vi "pickRobotsVSS.vi"(8 "error in (no error)":errorcluster, 11 "Game in":refnum<class "Game.lvclass">) -> (0 "error out":errorcluster, 3 "Game out":refnum<class "Game.lvclass">)   [LabVIEW 2018, in "Game.lvclass"]
uses:
  Game.lvclass
  Game.lvclass/Game.ctl
  Referee_class/Referee.lvclass/Referee.ctl
  Team_class/Team.lvclass/Team.ctl
  Robot_class/roles.ctl
  Robot_class/Robot.lvclass/Robot.ctl
  Role_class/Role.lvclass/Role.ctl
  HaltPlay_class/HaltPlay.lvclass/HaltPlay.ctl
  Playbook_class/Playbook.lvclass/Playbook.ctl
  ZigZagPlay_class/ZigZagPlay.lvclass/ZigZagPlay.ctl
  Robot_class/Robot.lvclass
  Playbook_class/Playbook.lvclass
  Ally_class/Ally.lvclass
  C:/Users/anton/Desktop/RoboIme/vsspssl/SSL_AI/Team_class/Team.lvclass
  Role_class/Write RobotRef.vi
  Robot_class/Write role.vi
  HaltPlay_class/Read Roles.vi
  HaltPlay_class/Write Roles.vi
  ZigZagPlay_class/Read Roles.vi
  ZigZagPlay_class/Write Roles.vi
  Playbook_class/Write keeper_plays.vi
  Playbook_class/Read keeper_plays.vi
  Read KeeperTeam.vi
  Read AllyRef.vi
  Read Referee.vi
  Read TestMode IDs.vi
  Referee_class/Read our_goalie_id.vi
  Team_class/Read RobotRef.vi
  Team_class/Write RobotRef.vi
  Write KeeperTeam.vi
  TimeoutRole_class/TimeoutRole.lvclass
  C:/Users/anton/Desktop/RoboIme/vsspssl/SSL_AI/Role_class/Role.lvclass
  HaltRole_class/HaltRole.lvclass
  ZigZagRole_class/ZigZagRole.lvclass
  Referee_class/Referee.lvclass
  PreparePenaltyAllyPlayVSS_class/PreparePenaltyAllyPlayVSS.lvclass
  HaltPlay_class/HaltPlay.lvclass
  DeadBallPlayVSS_class/DeadBallPlayVSS.lvclass
  NormalGamePlayVSS_class/NormalGamePlayVSS.lvclass
  BallChallengePlayVSS_class/BallChallengePlayVSS.lvclass
  PenaltyEnemyPlayVSS_class/PenaltyEnemyPlayVSS.lvclass
  TimeoutPlay_class/TimeoutPlay.lvclass
  Play_class/Play.lvclass
  TestPlay_class/TestPlay.lvclass
  KeeperPlay_class/KeeperPlay.lvclass
  ZigZagPlay_class/ZigZagPlay.lvclass
  GoToPlay_class/GoToPlay.lvclass
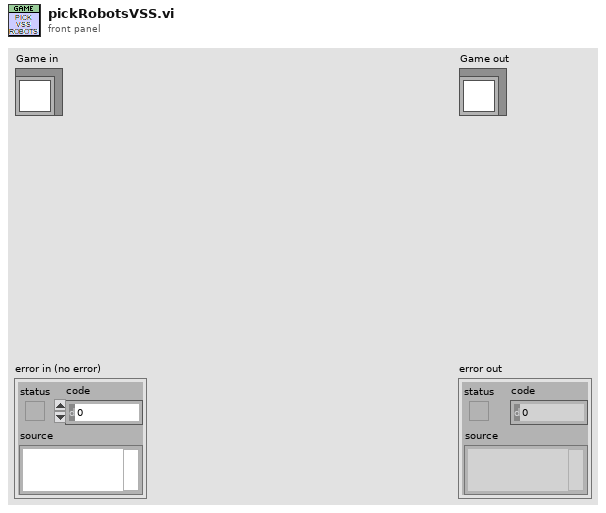
[diagram p1: front panel]
types:
  T1 = typedef "roles.ctl" = enum16{"Tabler", "TableFinalizer", "PrepareRollToPassRoller", "PrepareRollToPassReceiver", "SimplePassRoll", "SimplePassRollReceiver", "PenaltyDefense", "PreparePassReceiver 2", "PreparePassReceiver 1", "PassObserver", "Timeout", "Goto", "ZigZag", "None", "BallOutOfField", "DefenderArea", "Duelist", "AttackerStop", "FollowAttacker", "KeeperRole", "KickPenalty", "AttackerAimGoal", "AttackerBlock", "Marker", "Halt", "Shoot", "PassKicker", "PassReceiver", "TestRole", "PenaltyAttacker"}
  T2 = enum16{"Timeout", "DeadBall", "NormalGame", "KickPenaltyAlly", "PenaltyEnemy", "BallChallenge", "PreparePenaltyAlly", "Halt"}
  T3 = cluster{"PreparePenaltyAllyPlayVSS":refnum<class "PreparePenaltyAllyPlayVSS.lvclass">, "HaltPlay":refnum<class "HaltPlay.lvclass">, "DeadBallPlayVSS":refnum<class "DeadBallPlayVSS.lvclass">, "NormalGamePlayVSS":refnum<class "NormalGamePlayVSS.lvclass">, "BallChallengePlayVSS":refnum<class "BallChallengePlayVSS.lvclass">, "PenaltyEnemyPlayVSS":refnum<class "PenaltyEnemyPlayVSS.lvclass">, "TimeoutPlay":refnum<class "TimeoutPlay.lvclass">}
  T4 = cluster{"TimeoutRole 1":refnum<class "TimeoutRole.lvclass">}
  T5 = cluster{"HaltRole 1":refnum<class "HaltRole.lvclass">, "HaltRole 2":refnum<class "HaltRole.lvclass">, "HaltRole 3":refnum<class "HaltRole.lvclass">, "HaltRole 4":refnum<class "HaltRole.lvclass">, "HaltRole 5":refnum<class "HaltRole.lvclass">, "HaltRole 6":refnum<class "HaltRole.lvclass">}
  T6 = typedef "keeper_plays.ctl" = cluster{"Play":refnum<class "Play.lvclass">, "TestPlay":refnum<class "TestPlay.lvclass">, "HaltPlay":refnum<class "HaltPlay.lvclass">, "KeeperPlay":refnum<class "KeeperPlay.lvclass">, "TimeoutPlay":refnum<class "TimeoutPlay.lvclass">, "ZigZagPlay":refnum<class "ZigZagPlay.lvclass">, "GoToPlay":refnum<class "GoToPlay.lvclass">}
  T7 = cluster{"ZigZagRole":refnum<class "ZigZagRole.lvclass">}
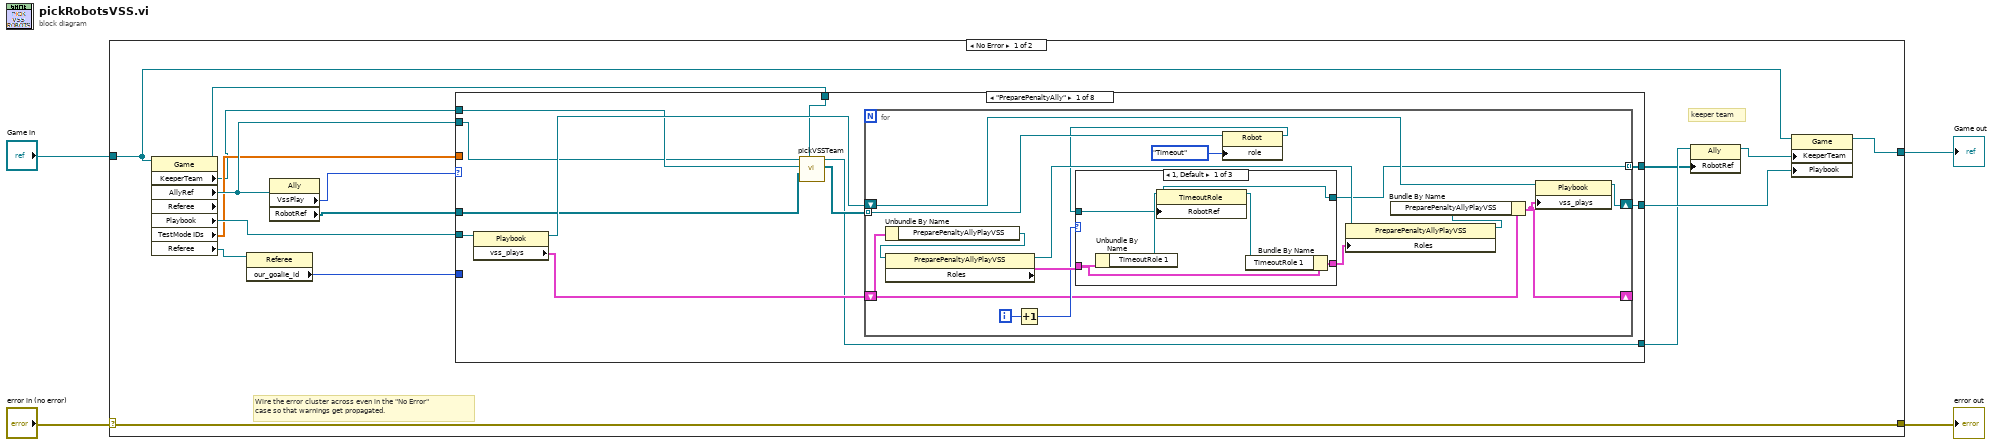
[diagram p0: block diagram]
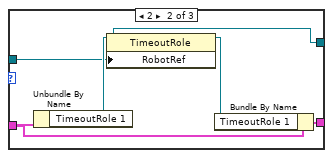
[diagram p2: hidden frame]
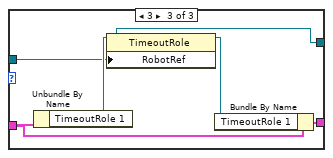
[diagram p3: hidden frame]
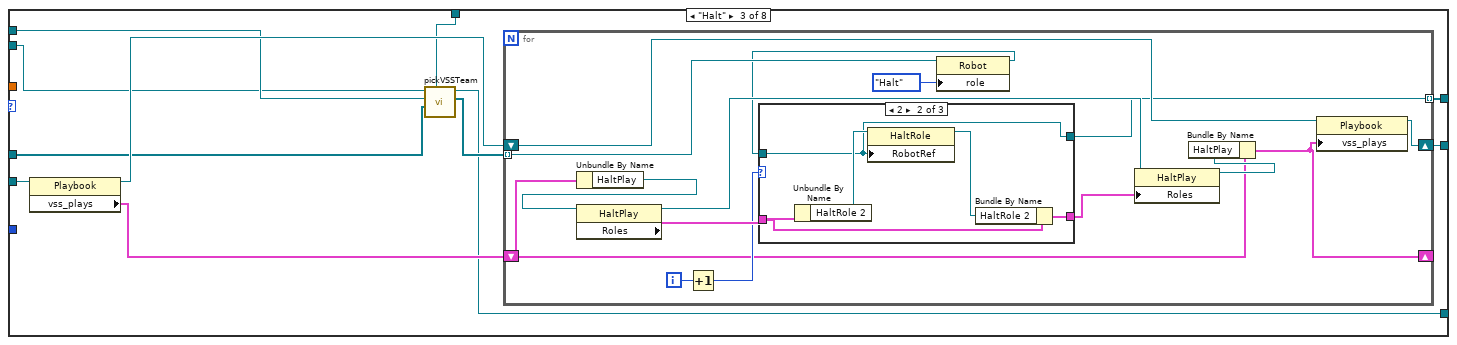
[diagram p5: hidden frame]
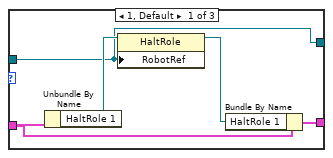
[diagram p6: hidden frame]
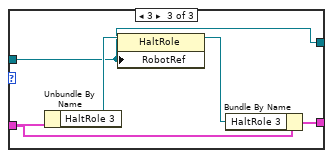
[diagram p7: hidden frame]
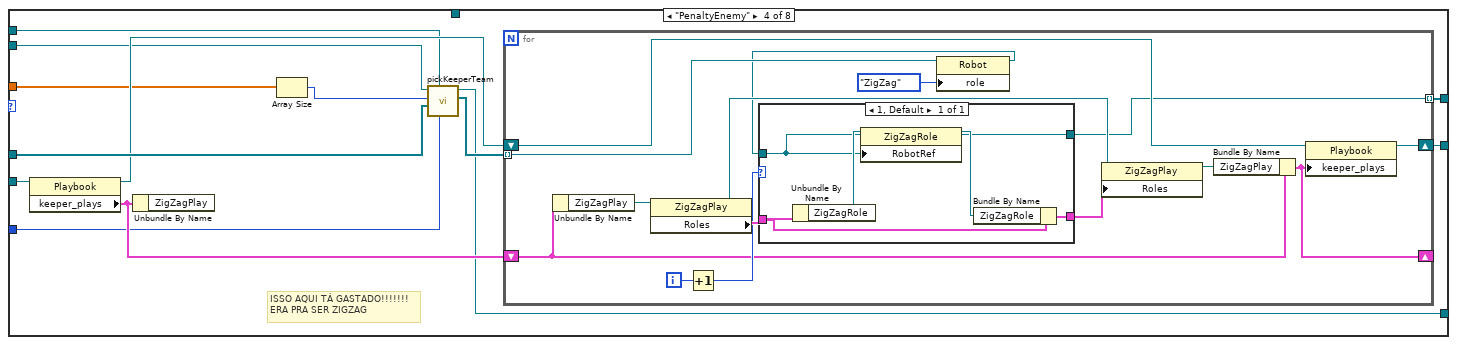
[diagram p8: hidden frame]
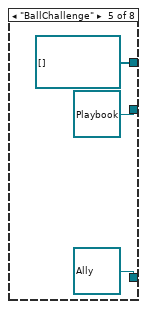
[diagram p9: hidden frame]
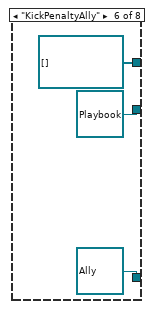
[diagram p10: hidden frame]
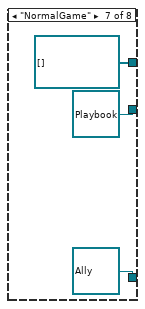
[diagram p11: hidden frame]
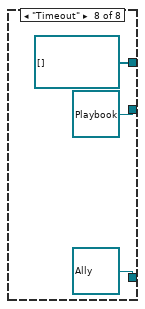
[diagram p12: hidden frame]
diagram:
  n1 = case shown="No Error" "error in (no error)" {
    selector: "error in (no error)" -> [w15 w149]
    tunnel: [w15 w149] -> w3
    tunnel: [w16 w148] -> w1
    tunnel: "Game in" -> [w18 w148]
    frame No Error {
      # "keeper team"
      # "Wire the error cluster across even in the \"No Error\"\ncase so that warnings get propagated."
      n2 = property class="Game" props=["KeeperTeam", "AllyRef", "Referee", "Playbook", "TestMode IDs", "Referee"](reference=w18) -> (reference out=w5:refnum<class "Game.lvclass">, "KeeperTeam"=w6:refnum<class "Ally.lvclass">, "AllyRef"=w12:refnum<class "Ally.lvclass">, "Playbook"=w20:refnum<class "Playbook.lvclass">, "TestMode IDs"=w9:dbl[], "Referee"=w8:refnum<class "Referee.lvclass">)  [unwired: 1 in, 2 out]
      n3 = property class="Referee"(reference=w8) -> ("our_goalie_id"=w7:i32)  [unwired: 1 in, 2 out]
      n4 = property class="Ally"(reference=w12) -> ("VssPlay"=w10:T2, "RobotRef"=w19:refnum<class "Robot.lvclass">[])  [unwired: 1 in, 2 out]
      n5 = case shown="\"PreparePenaltyAlly\"" w10 {
        tunnel: w20 -> [w31 _ w72 w115 _ _ _ _]
        tunnel: w19 -> [w24 _ w65 w111 _ _ _ _]
        tunnel: [w29 _ w70 w113 refnum<class "Playbook.lvclass"> refnum ("Playbook") refnum<class "Playbook.lvclass"> refnum ("Playbook") refnum<class "Playbook.lvclass"> refnum ("Playbook") refnum<class "Playbook.lvclass"> refnum ("Playbook")] -> w17
        tunnel: [w28 _ w69 w112 refnum<class "Robot.lvclass">[] [] refnum<class "Robot.lvclass">[] [] refnum<class "Robot.lvclass">[] [] refnum<class "Robot.lvclass">[] []] -> w11
        tunnel: [w21 _ w62 w108 refnum<class "Ally.lvclass"> refnum ("Ally out") refnum<class "Ally.lvclass"> refnum ("Ally out") refnum<class "Ally.lvclass"> refnum ("Ally out") refnum<class "Ally.lvclass"> refnum ("Ally out")] -> w13
        tunnel: w12 -> [w25 _ w66 w107 _ _ _ _]
        tunnel: w9 -> [_ _ _ w106 _ _ _ _]
        tunnel: w7 -> [_ _ _ w104 _ _ _ _]
        tunnel: w6 -> [w26 _ w67 w103 _ _ _ _]
        tunnel: w5 -> [w23 _ w64 _ _ _ _ _]
        frame "PreparePenaltyAlly" {
          n6 = property class="Playbook"(reference=w31) -> (reference out=w27:refnum<class "Playbook.lvclass">, "vss_plays"=w30:T3)  [unwired: 1 in, 1 out]
          n7 = call "pickVSSTeam.vi"("Ally in"=w25, "OldVSSTeam"=w26, "RobotRef"=w24, "Game"=w23) -> ("Ally out"=w21:refnum<class "Ally.lvclass">, "RobotRef Out"=w22:refnum<class "Robot.lvclass">[])  [unwired: 4 in, 1 out]
          n8 = for {
            tunnel: [w34] -> w28 mode=indexing
            tunnel: w22 -> [w39] mode=indexing
            shift-right: [w41] -> w29
            shift-left: w27 -> [w42]
            shift-right: [w32] -> _
            shift-left: w30 -> [w36]
            i -> [w38]
            n9 = Unbundle By Name(w36) -> ("PreparePenaltyAllyPlayVSS"=w35:refnum<class "PreparePenaltyAllyPlayVSS.lvclass">)
            n10 = property class="PreparePenaltyAllyPlayVSS"(reference=w35) -> (reference out=w44:refnum<class "PreparePenaltyAllyPlayVSS.lvclass">, "Roles"=w46:T4)  [unwired: 1 in, 1 out]
            n11 = Increment(x=w38) -> (x+1=w37:i32)
            n12 = property class="Robot"(reference=w39, "role"=roles."Timeout") -> (reference out=w33:refnum<class "Robot.lvclass">)  [unwired: 1 in, 1 out]
            n13 = case shown="1, Default" w37 {
              tunnel: w46 -> [w50 w55 w60]
              tunnel: [w49 w54 w59] -> w45
              tunnel: w33 -> [w47 w52 w57]
              tunnel: [w47 w52 w57] -> w34
              frame 1, Default {
                n14 = Unbundle By Name(w50) -> ("TimeoutRole 1"=w51:refnum<class "TimeoutRole.lvclass">)
                n15 = property class="TimeoutRole"(reference=w51, "RobotRef"=w47) -> (reference out=w48:refnum<class "TimeoutRole.lvclass">)  [unwired: 1 in, 1 out]
                n16 = Bundle By Name(cluster=w50, "TimeoutRole 1"=w48) -> (w49:T4)
              }
              frame 2 {
                n17 = Unbundle By Name(w55) -> ("TimeoutRole 1"=w56:refnum<class "TimeoutRole.lvclass">)
                n18 = property class="TimeoutRole"(reference=w56, "RobotRef"=w52) -> (reference out=w53:refnum<class "TimeoutRole.lvclass">)  [unwired: 1 in, 1 out]
                n19 = Bundle By Name(cluster=w55, "TimeoutRole 1"=w53) -> (w54:T4)
              }
              frame 3 {
                n20 = Unbundle By Name(w60) -> ("TimeoutRole 1"=w61:refnum<class "TimeoutRole.lvclass">)
                n21 = property class="TimeoutRole"(reference=w61, "RobotRef"=w57) -> (reference out=w58:refnum<class "TimeoutRole.lvclass">)  [unwired: 1 in, 1 out]
                n22 = Bundle By Name(cluster=w60, "TimeoutRole 1"=w58) -> (w59:T4)
              }
            }
            n23 = property class="PreparePenaltyAllyPlayVSS"(reference=w44, "Roles"=w45) -> (reference out=w43:refnum<class "PreparePenaltyAllyPlayVSS.lvclass">)  [unwired: 1 in, 1 out]
            n24 = Bundle By Name(cluster=w36, "PreparePenaltyAllyPlayVSS"=w43) -> (w32:T3)
            n25 = property class="Playbook"(reference=w42, "vss_plays"=w32) -> (reference out=w41:refnum<class "Playbook.lvclass">)  [unwired: 1 in, 1 out]
          }
        }
        frame "DeadBall" {
        }
        frame "Halt" {
          n26 = property class="Playbook"(reference=w72) -> (reference out=w68:refnum<class "Playbook.lvclass">, "vss_plays"=w71:T3)  [unwired: 1 in, 1 out]
          n27 = call "pickVSSTeam.vi"("Ally in"=w66, "OldVSSTeam"=w67, "RobotRef"=w65, "Game"=w64) -> ("Ally out"=w62:refnum<class "Ally.lvclass">, "RobotRef Out"=w63:refnum<class "Robot.lvclass">[])  [unwired: 4 in, 1 out]
          n28 = for {
            tunnel: [w75] -> w69 mode=indexing
            tunnel: w63 -> [w80] mode=indexing
            shift-right: [w82] -> w70
            shift-left: w68 -> [w83]
            shift-right: [w73] -> _
            shift-left: w71 -> [w77]
            i -> [w79]
            n29 = Unbundle By Name(w77) -> ("HaltPlay"=w76:refnum<class "HaltPlay.lvclass">)
            n30 = property class="HaltPlay"(reference=w76) -> (reference out=w85:refnum<class "HaltPlay.lvclass">, "Roles"=w87:T5)  [unwired: 1 in, 1 out]
            n31 = Increment(x=w79) -> (x+1=w78:i32)
            n32 = property class="Robot"(reference=w80, "role"=roles."Halt") -> (reference out=w74:refnum<class "Robot.lvclass">)  [unwired: 1 in, 1 out]
            n33 = case shown="2" w78 {
              tunnel: w87 -> [w91 w96 w101]
              tunnel: [w90 w95 w100] -> w86
              tunnel: w74 -> [w88 w93 w98]
              tunnel: [w88 w93 w98] -> w75
              frame 1, Default {
                n34 = Unbundle By Name(w91) -> ("HaltRole 1"=w92:refnum<class "HaltRole.lvclass">)
                n35 = property class="HaltRole"(reference=w92, "RobotRef"=w88) -> (reference out=w89:refnum<class "HaltRole.lvclass">)  [unwired: 1 in, 1 out]
                n36 = Bundle By Name(cluster=w91, "HaltRole 1"=w89) -> (w90:T5)
              }
              frame 2 {
                n37 = Unbundle By Name(w96) -> ("HaltRole 2"=w97:refnum<class "HaltRole.lvclass">)
                n38 = property class="HaltRole"(reference=w97, "RobotRef"=w93) -> (reference out=w94:refnum<class "HaltRole.lvclass">)  [unwired: 1 in, 1 out]
                n39 = Bundle By Name(cluster=w96, "HaltRole 2"=w94) -> (w95:T5)
              }
              frame 3 {
                n40 = Unbundle By Name(w101) -> ("HaltRole 3"=w102:refnum<class "HaltRole.lvclass">)
                n41 = property class="HaltRole"(reference=w102, "RobotRef"=w98) -> (reference out=w99:refnum<class "HaltRole.lvclass">)  [unwired: 1 in, 1 out]
                n42 = Bundle By Name(cluster=w101, "HaltRole 3"=w99) -> (w100:T5)
              }
            }
            n43 = property class="HaltPlay"(reference=w85, "Roles"=w86) -> (reference out=w84:refnum<class "HaltPlay.lvclass">)  [unwired: 1 in, 1 out]
            n44 = Bundle By Name(cluster=w77, "HaltPlay"=w84) -> (w73:T3)
            n45 = property class="Playbook"(reference=w83, "vss_plays"=w73) -> (reference out=w82:refnum<class "Playbook.lvclass">)  [unwired: 1 in, 1 out]
          }
        }
        frame "PenaltyEnemy" {
          # "ISSO AQUI TÁ GASTADO!!!!!!!\nERA PRA SER ZIGZAG"
          n46 = property class="Playbook"(reference=w115) -> (reference out=w110:refnum<class "Playbook.lvclass">, "keeper_plays"=w114:T6)  [unwired: 1 in, 1 out]
          n47 = Unbundle By Name(w114) -> ()  [unwired: 1 out]
          n48 = Array Size(array=w106) -> (size(s)=w105:i32)
          n49 = call-dynamic "pickKeeperTeam.vi"("our_goalie_id"=w104, "OldKepperTeam"=w103, "RobotRef"=w111, "NumberOfRobots"=w105, "Ally in"=w107) -> ("RobotRef out"=w109:refnum<class "Robot.lvclass">[], "Ally out"=w108:refnum<class "Ally.lvclass">)  [unwired: 4 in, 1 out]
          n50 = for {
            tunnel: [w116] -> w112 mode=indexing
            tunnel: w109 -> [w123] mode=indexing
            shift-right: [w125] -> w113
            shift-left: w110 -> [w126]
            shift-right: [w120] -> _
            shift-left: w114 -> [w119]
            i -> [w122]
            n51 = Unbundle By Name(w119) -> ("ZigZagPlay"=w118:refnum<class "ZigZagPlay.lvclass">)
            n52 = property class="ZigZagPlay"(reference=w118) -> (reference out=w128:refnum<class "ZigZagPlay.lvclass">, "Roles"=w130:T7)  [unwired: 1 in, 1 out]
            n53 = Increment(x=w122) -> (x+1=w121:i32)
            n54 = property class="Robot"(reference=w123, "role"=roles."ZigZag") -> (reference out=w117:refnum<class "Robot.lvclass">)  [unwired: 1 in, 1 out]
            n55 = case shown="1, Default" w121 {
              tunnel: w130 -> [w134]
              tunnel: [w133] -> w129
              tunnel: w117 -> [w131]
              tunnel: [w131] -> w116
              frame 1, Default {
                n56 = Unbundle By Name(w134) -> ("ZigZagRole"=w135:refnum<class "ZigZagRole.lvclass">)
                n57 = property class="ZigZagRole"(reference=w135, "RobotRef"=w131) -> (reference out=w132:refnum<class "ZigZagRole.lvclass">)  [unwired: 1 in, 1 out]
                n58 = Bundle By Name(cluster=w134, "ZigZagRole"=w132) -> (w133:T7)
              }
            }
            n59 = property class="ZigZagPlay"(reference=w128, "Roles"=w129) -> (reference out=w127:refnum<class "ZigZagPlay.lvclass">)  [unwired: 1 in, 1 out]
            n60 = Bundle By Name(cluster=w119, "ZigZagPlay"=w127) -> (w120:T6)
            n61 = property class="Playbook"(reference=w126, "keeper_plays"=w120) -> (reference out=w125:refnum<class "Playbook.lvclass">)  [unwired: 1 in, 1 out]
          }
        }
        frame "BallChallenge" {
        }
        frame "KickPenaltyAlly" {
        }
        frame "NormalGame" {
        }
        frame "Timeout" {
        }
      }
      n62 = property class="Ally"(reference=w13, "RobotRef"=w11) -> (reference out=w14:refnum<class "Ally.lvclass">)  [unwired: 1 in, 1 out]
      n63 = property class="Game"(reference=w18, "KeeperTeam"=w14, "Playbook"=w17) -> (reference out=w16:refnum<class "Game.lvclass">)  [unwired: 1 in, 1 out]
    }
    frame Error {
    }
  }
  "error out" <- w3
  "Game out" <- w1
